vi "Build.vi"(9 "XYZTheta":dbl[](array[numeric]), 10 "Pattern Coordinates":dbl[][](array[numeric]), 11 "CAD Dispense2 in":refnum<class "CAD Dispense2.lvclass">) -> (1 "Starting Coordinates":dbl[](array[numeric]), 3 "CAD Dispense2 out":refnum<class "CAD Dispense2.lvclass">)   [LabVIEW 2016, in "CAD Dispense2.lvclass"]
uses:
  CAD Dispense2.lvclass
  D:/UCSB-Gantry 0418/V5/Classes/Routine/Dispense/Dispense.lvclass
  Dispense.lvclass/Dispense.ctl
  CAD Dispense2.lvclass/CAD Dispense2.ctl
  <vilib>/Analysis/coordinate.llb/2D Cartesian Coordinate Rotation (Scalar).vi
  Read Z Height.vi
  <vilib>/Analysis/NI_AALPro.lvlib
panel:
  out "xy1,xy2":dbl[][](array[numeric])
  out "centers":dbl[][](array[numeric])
  out "xy1,xy2,...":dbl[][](array[numeric])
  out "CW/CCW":dbl[](array[numeric])
  out "Cell Count":dbl[](array[numeric])
  out "data":T1(array[cluster])
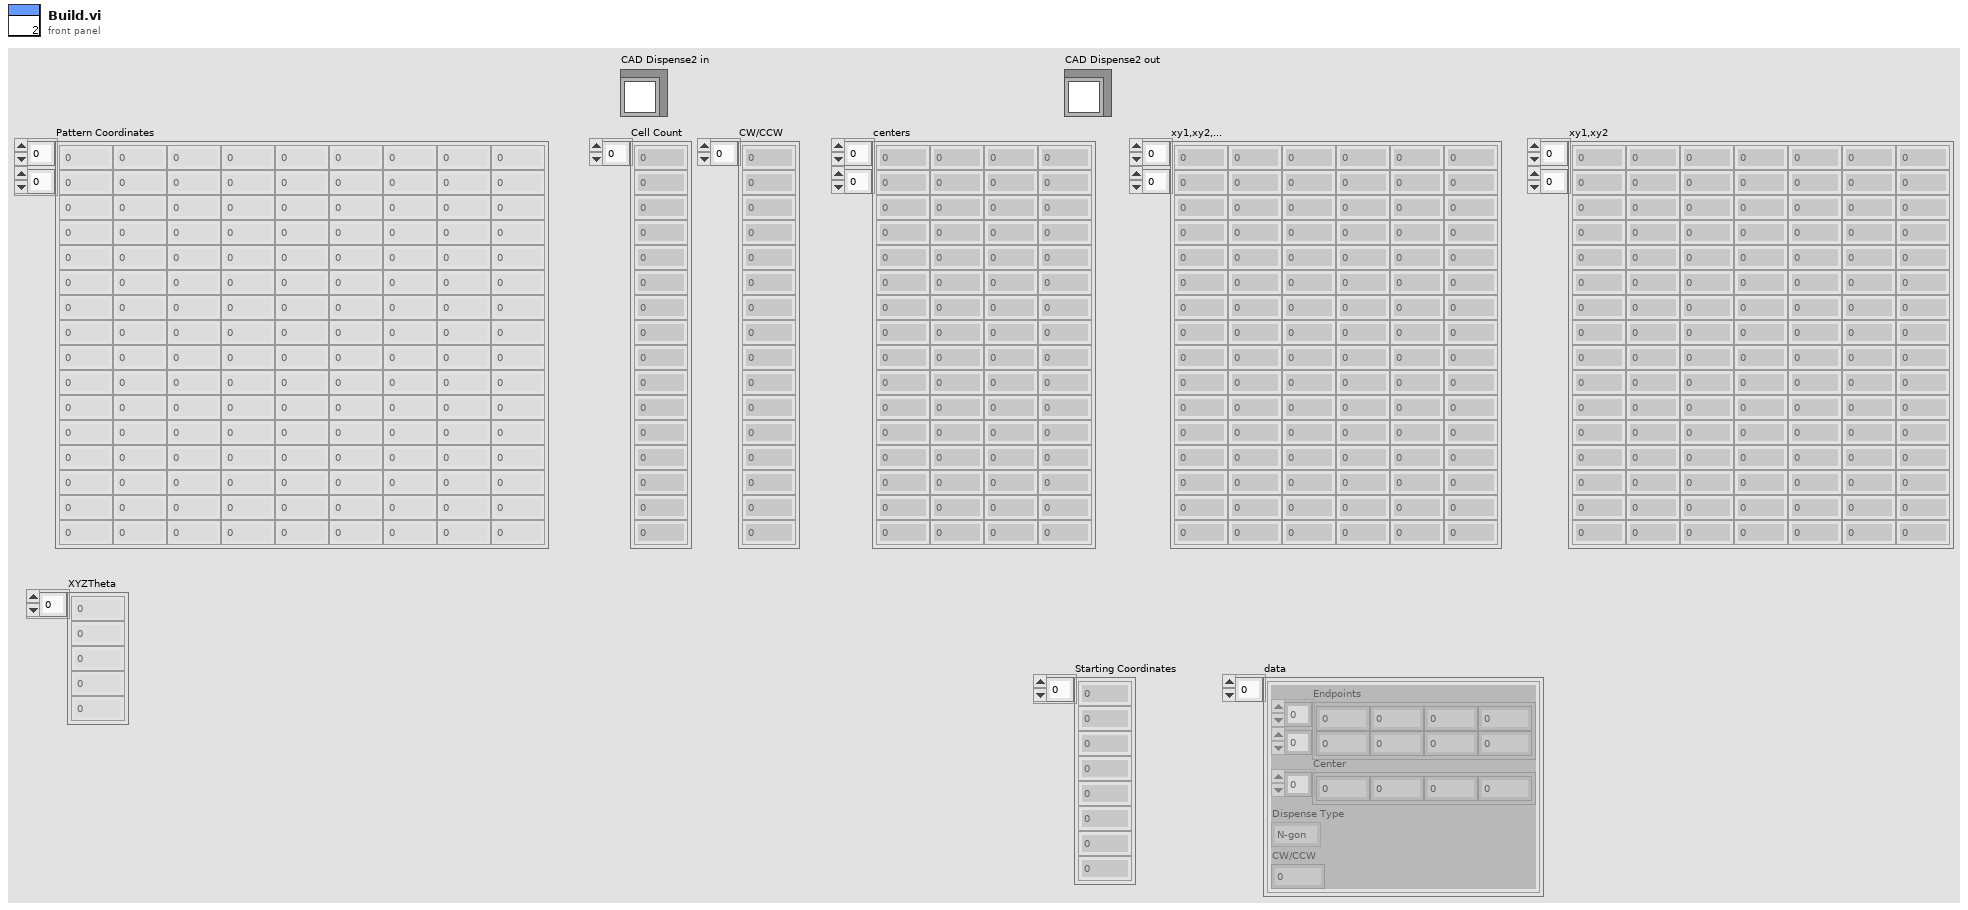
[diagram p1: front panel]
types:
  T1 = cluster{"Endpoints":dbl[][], "Center":dbl[], "Dispense Type":enum16{"N-gon", "Square", "Arc", "Dot", "Line", "Circle"}, "CW/CCW":dbl}[]
  T2 = enum16{"N-gon", "Square", "Arc", "Dot", "Line", "Circle"}
  T3 = cluster{"Endpoints":dbl[][], "Center":dbl[], "Dispense Type":enum16{"N-gon", "Square", "Arc", "Dot", "Line", "Circle"}, "CW/CCW":dbl}
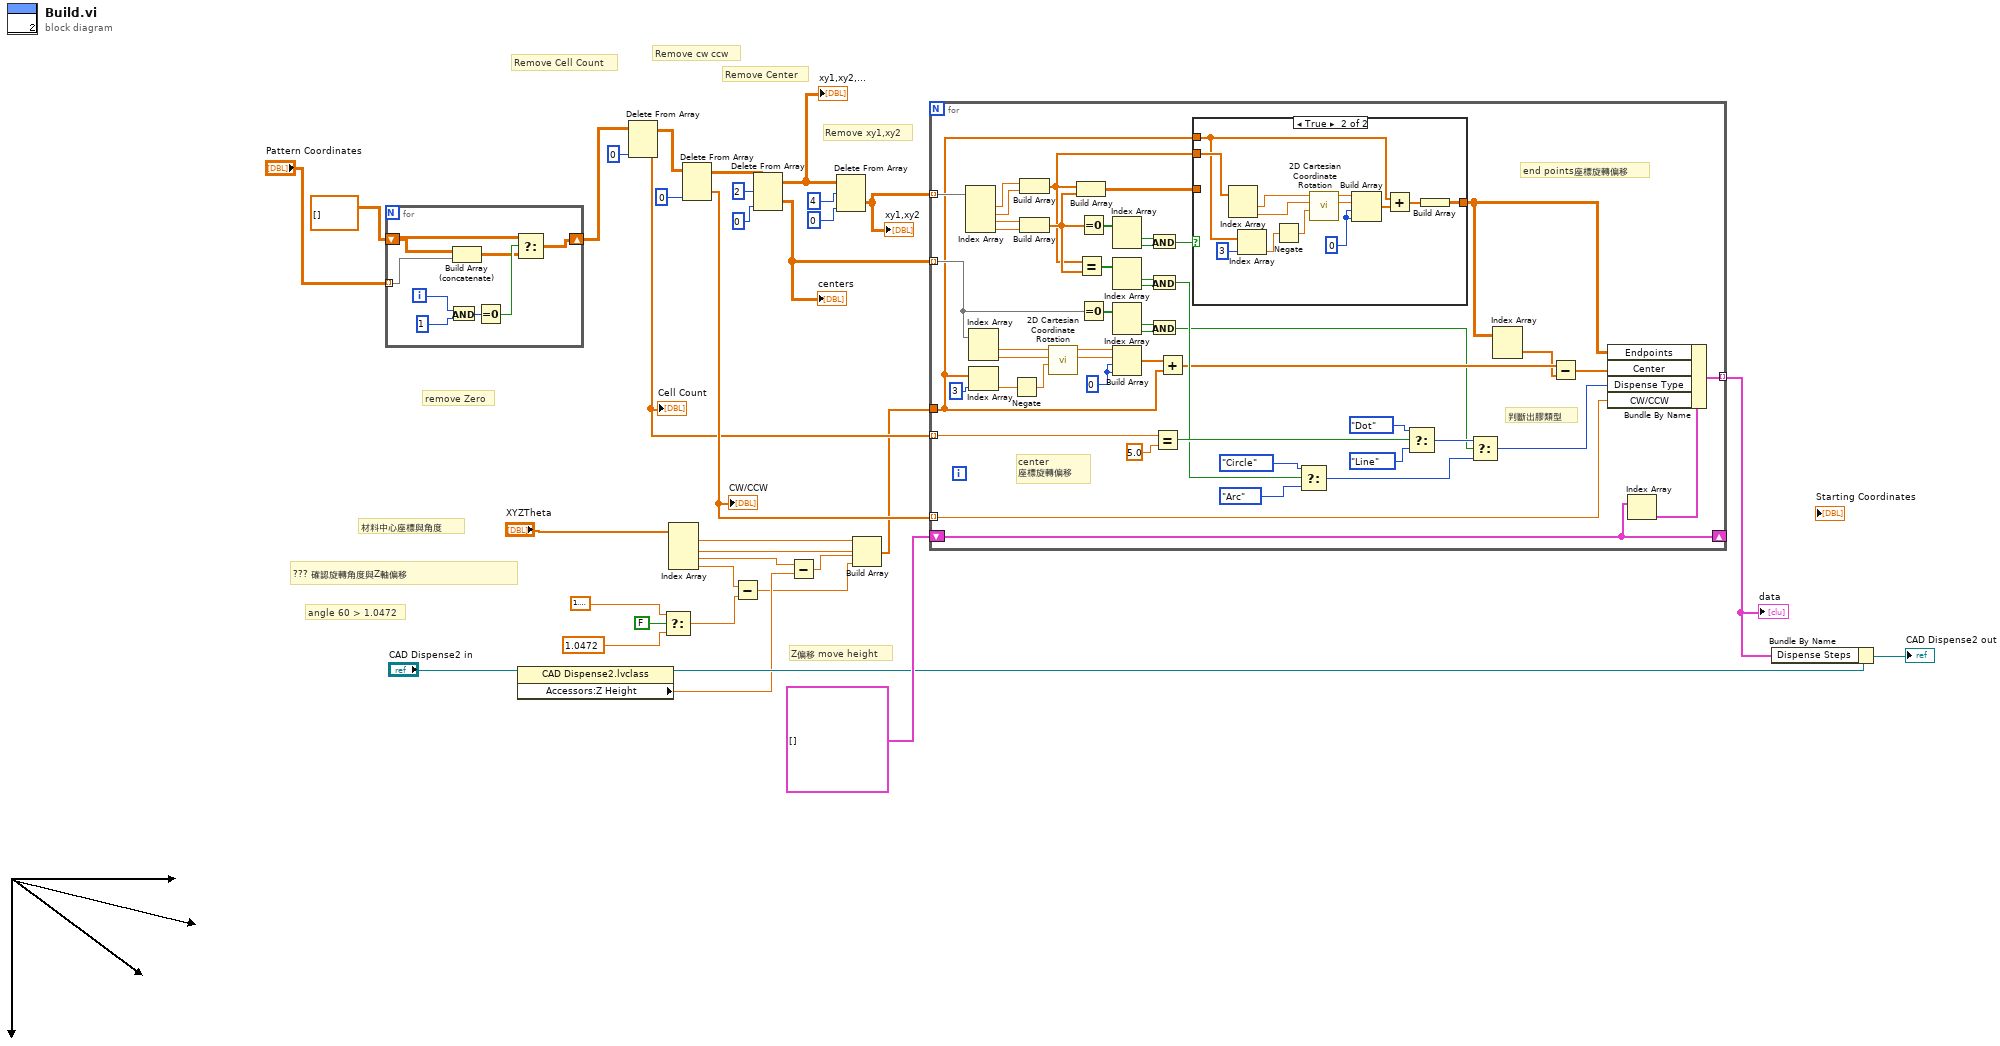
[diagram p0: block diagram]
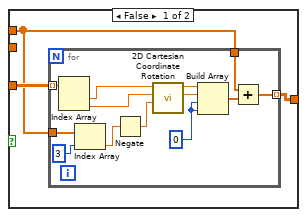
[diagram p2: hidden frame]
diagram:
  # "angle 60 > 1.0472"
  # "Remove xy1,xy2"
  # "材料中心座標與角度"
  # "Z偏移 move height"
  # "remove Zero"
  # "??? 確認旋轉角度與Z軸偏移"
  # "Remove Center"
  # "Remove cw ccw"
  # "Remove Cell Count"
  n1 = for {
    shift-right: [w36] -> w21
    shift-left: dbl[][] [] -> [w38]
    tunnel: "Pattern Coordinates" -> [w39] mode=indexing
    i -> [w40]
    n2 = And(x=w40, y=1 ("x")) -> (x .and. y?=w41:i32)
    n3 = Build Array (concatenate)(w38, w39) -> (w35:dbl[][])
    n4 = Equal To 0?(x=w41) -> (x = 0?=w37:bool)
    n5 = Select(t=w38, s=w37, f=w35) -> (s? t:f=w36:dbl[][])
  }
  n6 = property class="CAD Dispense2.lvclass"(reference="CAD Dispense2 in") -> (reference out=w30:refnum<class "CAD Dispense2.lvclass">, "Accessors:Z Height"=w16:dbl)  [unwired: 1 in, 1 out]
  n7 = Delete From Array "Delete From Array"(array=w21, index (col)=0 ("disabled index (col)")) -> (deleted portion=w19:dbl[], array with subset deleted=w27:dbl[][])  [unwired: 2 in]
  "Cell Count" <- w19
  n8 = Select(t=1.5707963267948966, s=FALSE, f=1.0472 ("theta")) -> (s? t:f=w3:dbl)
  n9 = Index Array(array="XYZTheta") -> (element #1=w15:dbl, element #2=w14:dbl, element #3=w17:dbl, element #4=w18:dbl)  [unwired: 4 in]
  n10 = Delete From Array(array=w27, index (col)=0 ("disabled index (col)")) -> (deleted portion=w20:dbl[], array with subset deleted=w24:dbl[][])  [unwired: 2 in]
  "CW/CCW" <- w20
  n11 = Subtract(x=w18, y=w3) -> (x-y=w12:dbl)
  n12 = Delete From Array(array=w24, length=2, index (col)=0 ("disabled index (col)")) -> (deleted portion=w10:dbl[][], array with subset deleted=w9:dbl[][])  [unwired: 1 in]
  "xy1,xy2,..." <- w9
  "centers" <- w10
  n13 = Subtract(x=w17, y=w16) -> (x-y=w13:dbl)
  n14 = Delete From Array(array=w9, length=4, index (col)=0 ("disabled index (col)")) -> (deleted portion=w6:dbl[][])  [unwired: 1 in, 1 out]
  "xy1,xy2" <- w6
  n15 = Build Array(w15, w14, w13, w12) -> (w11:dbl[])
  n16 = for {
    shift-right: [w91] -> _
    shift-left: T1 [] ("Coordinates.CAD Cluster") -> [w91]
    tunnel: [w89] -> w32 mode=indexing
    tunnel: w20 -> [w88] mode=indexing
    tunnel: w19 -> [w69] mode=indexing
    tunnel: w11 -> [w43]
    tunnel: w10 -> [w46] mode=indexing
    tunnel: w6 -> [w87] mode=indexing
    w56 = 0
    # "center \n座標旋轉偏移"
    # "end points座標旋轉偏移"
    # "判斷出膠類型"
    n17 = Index Array(array=w87) -> (element #1=w83:dbl, element #2=w82:dbl, element #3=w81:dbl, element #4=w80:dbl)  [unwired: 4 in]
    n18 = Index Array(array=w46) -> (element #1=w85:dbl, element #2=w84:dbl)  [unwired: 2 in]
    n19 = Index Array(array=w43, index=3) -> (element=w54:dbl)
    n20 = Negate(x=w54) -> (-x=w86:dbl)
    n21 = Build Array(w83, w82) -> (w78:dbl[])
    n22 = Build Array(w81, w80) -> (w79:dbl[])
    n23 = call-poly <vilib>:"2D Cartesian Coordinate Rotation.vi"("theta"=w86, "y"=w84, "x"=w85) -> ("y out"=w57:dbl, "x out"=w58:dbl)  [unwired: 6 in, 1 out]
    n24 = Build Array(w78, w79) -> (w77:dbl[][])
    n25 = Equal?(x=w78, y=w79) -> (x = y?=w70:bool[])
    n26 = Equal To 0?(x=w79) -> (x = 0?=w76:bool[])
    n27 = Equal To 0?(x=w46) -> (x = 0?=w47:bool[])
    n28 = Index Array(array=w76) -> (element #1=w74:bool, element #2=w75:bool)  [unwired: 2 in]
    n29 = Index Array(array=w70) -> (element #1=w72:bool, element #2=w71:bool)  [unwired: 2 in]
    n30 = Index Array(array=w47) -> (element #1=w49:bool, element #2=w48:bool)  [unwired: 2 in]
    n31 = Build Array(w58, w57, w56, w56) -> (w44:dbl[])
    n32 = And(x=w74, y=w75) -> (x .and. y?=w73:bool)
    n33 = And(x=w72, y=w71) -> (x .and. y?=w64:bool)
    n34 = And(x=w49, y=w48) -> (x .and. y?=w45:bool)
    n35 = Equal?(x=w69, y=5.0) -> (x = y?=w66:bool)
    n36 = Add(x=w44, y=w43) -> (x+y=w52:dbl[])
    n37 = case shown="True" w73 {
      tunnel: w78 -> [_ w112]
      tunnel: w77 -> [w94 _]
      tunnel: w43 -> [w92 w111]
      tunnel: [w93 w108] -> w50
      frame False {
        n38 = for {
          tunnel: w94 -> [w107] mode=indexing
          tunnel: w92 -> [w100]
          tunnel: [w98] -> w93 mode=indexing
          tunnel: w92 -> [w96]
          w106 = 0
          n39 = Index Array(array=w107) -> (element #1=w102:dbl, element #2=w101:dbl)  [unwired: 2 in]
          n40 = Index Array(array=w96, index=3) -> (element=w95:dbl)
          n41 = Negate(x=w95) -> (-x=w103:dbl)
          n42 = call-poly <vilib>:"2D Cartesian Coordinate Rotation.vi"("theta"=w103, "y"=w101, "x"=w102) -> ("y out"=w105:dbl, "x out"=w104:dbl)  [unwired: 6 in, 1 out]
          n43 = Build Array(w104, w105, w106, w106) -> (w99:dbl[])
          n44 = Add(x=w100, y=w99) -> (x+y=w98:dbl[])
        }
      }
      frame True {
        w120 = 0
        n45 = Index Array(array=w112) -> (element #1=w116:dbl, element #2=w115:dbl)  [unwired: 2 in]
        n46 = Index Array(array=w111, index=3) -> (element=w110:dbl)
        n47 = Negate(x=w110) -> (-x=w117:dbl)
        n48 = call-poly <vilib>:"2D Cartesian Coordinate Rotation.vi"("theta"=w117, "y"=w115, "x"=w116) -> ("y out"=w119:dbl, "x out"=w118:dbl)  [unwired: 6 in, 1 out]
        n49 = Build Array(w118, w119, w120, w120) -> (w114:dbl[])
        n50 = Add(x=w111, y=w114) -> (x+y=w109:dbl[])
        n51 = Build Array(w109) -> (w108:dbl[][])
      }
    }
    n52 = Select(t=T2."Circle" ("Dispense Type"), s=w64, f=T2."Arc" ("Dispense Type")) -> (s? t:f=w65:T2)
    n53 = Select(t=T2."Dot" ("Dispense Type"), s=w66, f=T2."Line" ("Dispense Type")) -> (s? t:f=w67:T2)
    n54 = Select(t=w67, s=w45, f=w65) -> (s? t:f=w59:T2)
    n55 = Index Array(array=w50) -> (element=w51:dbl[])  [unwired: 2 in]
    n56 = Subtract(x=w52, y=w51) -> (x-y=w53:dbl[])
    n57 = Index Array(array=w91) -> (element=w90:T3)  [unwired: 1 in]
    n58 = Bundle By Name(cluster=w90, "Endpoints"=w50, "Center"=w53, "Dispense Type"=w59, "CW/CCW"=w88) -> (w89:T3)
  }
  "data" <- w32
  n59 = Bundle By Name(cluster=w30, "Dispense Steps"=w32) -> (→"CAD Dispense2 out":refnum<class "CAD Dispense2.lvclass">)
